vi "Match Block Upload Response.vi"(8 "error in":errorcluster, 10 "Frame Data":u8[](array[numeric]), 11 "Block Upload Initiate in":refnum<class "Block Upload Initiate Transfer.lvclass">) -> (0 "error out":errorcluster, 1 "SDO Result":T1={"Success"=FALSE, "SDO abort code"={"Null"=TRUE, "Value"=84082688}, "Data"={"Null"=TRUE, "Data"=[]}} {"SDO abort code"."Value" items=["Toggle bit not allowed"=84082688, "SDO protocol timed out"=84148224, "Client/server command specifier not valid or unknown"=84148225, "Invalid block size (block mode only)"=84148226, "Invalid sequence number (block mode only)"=84148227, "CRC error (block mode only)"=84148228, "Out of memory"=84148229, "Attempt to read a write only object"=100728833, "Attempt to write a read only object"=100728834, "Object does not exist in the object dictionary"=100794368, "Object cannot be mapped to the PDO"=100925505, "The number and length of the objects to be mapped would exceed PDO length"=100925506, "General parameter incompatibility reason"=100925507, "General internal incompatibility in the device"=100925511, "Access failed due to an hardware error"=101056512, "Data type does not match, length of service parameter does not match"=101122064, "Data type does not match, length of service parameter too high"=101122066, "Data type does not match, length of service parameter too low"=101122067, "Sub-index does not exist"=101253137, "Invalid value for parameter (download only)"=101253168, "Value of parameter written too high (download only)"=101253169, "Value of parameter written too low (download only)"=101253170, "Maximum value is less than minimum value"=101253174, "Resource not available: SDO connection"=101318691, "General error"=134217728, "Data cannot be transferred or stored to the application"=134217760, "Data cannot be transferred or stored to the application because of local control"=134217761, "Data cannot be transferred or stored to the application because of the present device stable"=134217762, "Object dictionary dynamic generation fails or no object dictionary is present (e.g. object dictionary is generated from file and generation fails because of an file error)"=134217763, "No data available"=134217764]; "Data"."Data" format="%02x"}, 2 "Match":bool, 3 "SDO Transfer out":refnum<class "SDO Transfer.lvclass">)   [LabVIEW 2020, in "CANopen.lvlib" / "SDO Manager.lvlib" / "Block Upload Initiate Transfer.lvclass"]
uses:
  Block Upload Initiate Transfer.lvclass
  Block Upload Initiate Transfer.lvclass/Block Upload Initiate Transfer.ctl
  D:/git/CANopen-LabVIEW/source/SDO Manager/SDO Manager/SDO Transfer/SDO Transfer.lvclass
  D:/git/CANopen-LabVIEW/source/Response Matcher/IResponse/IMatch Response.lvclass
  D:/git/CANopen-LabVIEW/source/SDO Manager/SDO Manager/Block Upload Initiate Transfer/Block Upload Initiate Transfer.lvclass
  Block Upload Sub-Block Transfer/Block Upload Sub-Block Transfer.lvclass
  D:/git/CANopen-LabVIEW/source/SDO Manager/SDO Manager/Block Upload Sub-Block Transfer/Block Upload Sub-Block Transfer.lvclass
  SDO Transfer/SDO Transfer.lvclass
  SDO Transfer/SDO abort code.ctl
  Typedefs/SDO Result.ctl
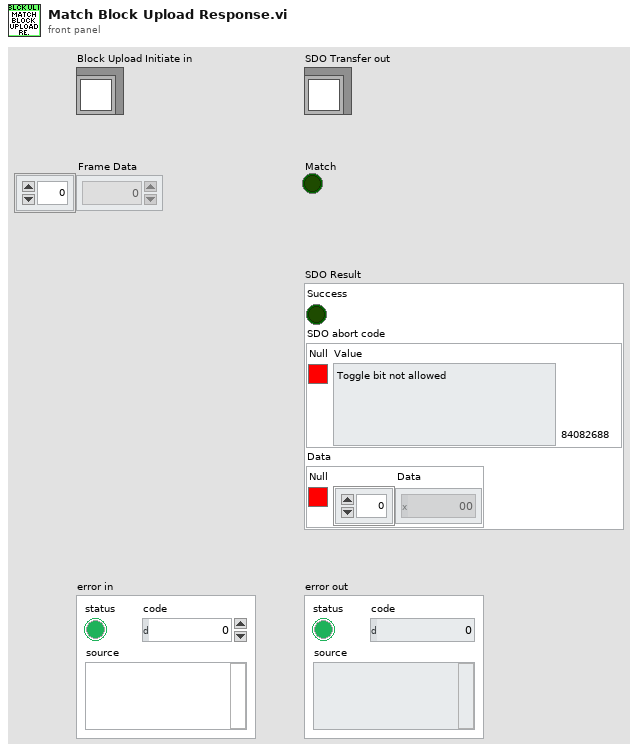
[diagram p1: front panel]
types:
  T1 = typedef "CANopen.lvlib/SDO Manager.lvlib/SDO Transfer.lvclass/SDO Result.ctl" = cluster{"Success":bool, "SDO abort code":cluster{"Null":bool, "Value":T2}, "Data":cluster{"Null":bool, "Data":u8[]}}
  T2 = typedef "CANopen.lvlib/SDO Manager.lvlib/SDO Transfer.lvclass/SDO abort code.ctl" = u32
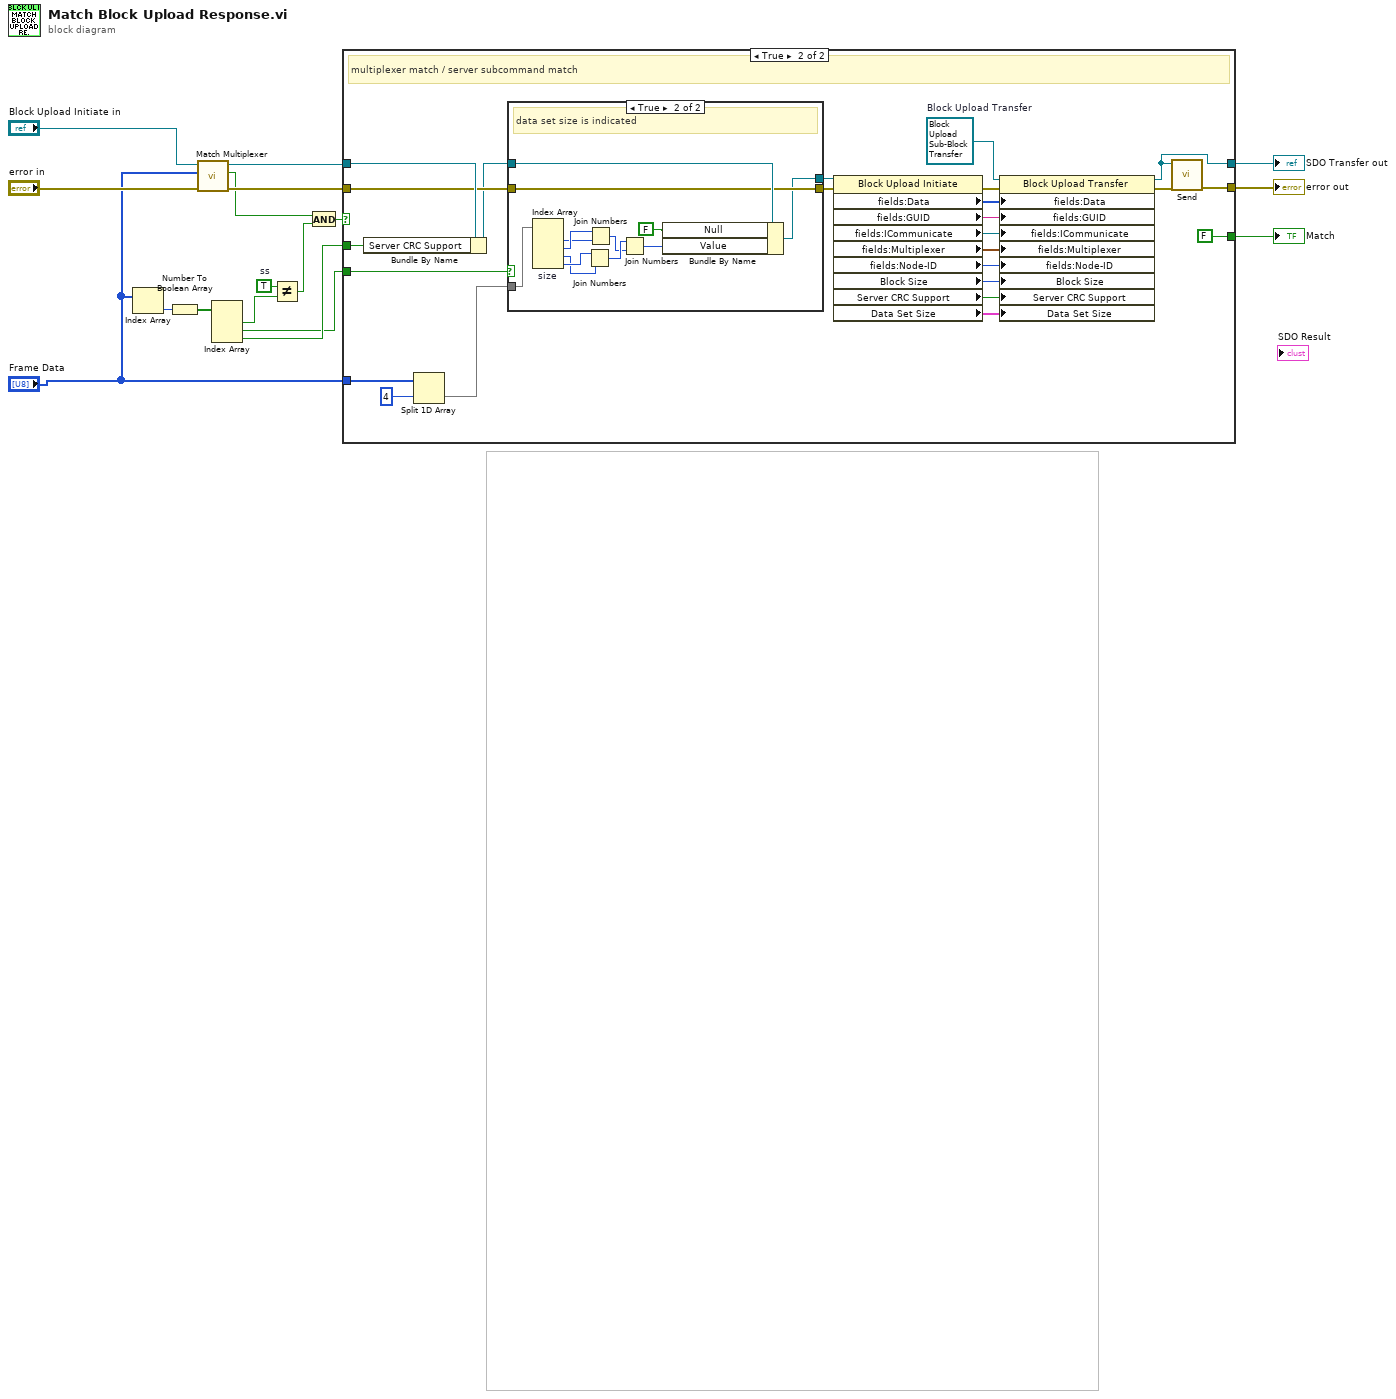
[diagram p0: block diagram]
diagram:
  w14 = TRUE  # ss
  n1 = Index Array(array="Frame Data") -> (element=w2:u8)  [unwired: 1 in]
  n2 = Number To Boolean Array(number=w2) -> (Boolean array=w12:bool[])
  n3 = call "Match Multiplexer.vi"("error in"="error in", "Frame Data"="Frame Data", "SDO Transfer in"="Block Upload Initiate in") -> ("error out"=w6:errorcluster, "Match"=w3:bool, "SDO Transfer out"=w4:refnum<class "Block Upload Initiate Transfer.lvclass">)  [unwired: 6 in]
  n4 = Index Array(array=w12) -> (element #1=w17:bool, element #2=w15:bool, element #3=w16:bool)  [unwired: 3 in]
  n5 = Not Equal?(x=w14, y=w17) -> (x != y?=w13:bool)
  n6 = And(x=w3, y=w13) -> (x .and. y?=w11:bool)
  n7 = case shown="True" w11 {
    tunnel: w6 -> [w19 w42]
    tunnel: w4 -> [w18 w43]
    tunnel: [w18 w20] -> w8
    tunnel: [w19 w28] -> w9
    tunnel: [_ FALSE] -> w10
    tunnel: w15 -> [_ w40]
    tunnel: w16 -> [_ w39]
    tunnel: "Frame Data" -> [_ w25]
    frame False {
      # "no match"
    }
    frame True {
      w37 = refnum<class "Block Upload Sub-Block Transfer.lvclass"> refnum  # Block Upload Transfer
      # "multiplexer match / server subcommand match"
      n8 = Bundle By Name(cluster=w43, "Server CRC Support"=w39) -> (w41:refnum<class "Block Upload Initiate Transfer.lvclass">)
      n9 = Split 1D Array(array=w25, index=4) -> (second subarray=w24:u8[])  [unwired: 1 out]
      n10 = case shown="True" w40 {
        tunnel: w24 -> [_ w55]
        tunnel: w41 -> [w44 w50]
        tunnel: w42 -> [w45 w48]
        tunnel: [w44 w47] -> w35
        tunnel: [w45 w48] -> w36
        frame False {
          # "data set size is not indicated"
        }
        frame True {
          # "data set size is indicated"
          n11 = Index Array "size"(array=w55) -> (element #1=w51:u8, element #2=w52:u8, element #3=w53:u8, element #4=w54:u8)  [unwired: 4 in]
          n12 = Join Numbers(hi=w54, lo=w53) -> ((hi.lo)=w57:u16)
          n13 = Join Numbers(hi=w52, lo=w51) -> ((hi.lo)=w56:u16)
          n14 = Join Numbers(hi=w57, lo=w56) -> ((hi.lo)=w46:u32)
          n15 = Bundle By Name(cluster=w50, "Null"=FALSE ("Data Set Size.Null"), "Value"=w46) -> (w47:refnum<class "Block Upload Initiate Transfer.lvclass">)
        }
      }
      n16 = property class="Block Upload Initiate"(reference=w35, error in=w36) -> (error out=w34:errorcluster, "fields:Data"=w22:u8[], "fields:GUID"=w30:string, "fields:ICommunicate"=w31:refnum<class "ICommunicate.lvclass">, "fields:Multiplexer"=w32:cluster{"Index":u16, "Sub-Index":u8}, "fields:Node-ID"=w33:u8, "Block Size"=w27:u8, "Server CRC Support"=w23:bool, "Data Set Size"=w21:cluster{"Null":bool, "Value":u32})  [unwired: 1 out]
      n17 = property class="Block Upload Transfer"(reference=w37, error in=w34, "fields:Data"=w22, "fields:GUID"=w30, "fields:ICommunicate"=w31, "fields:Multiplexer"=w32, "fields:Node-ID"=w33, "Block Size"=w27, "Server CRC Support"=w23, "Data Set Size"=w21) -> (reference out=w20:refnum<class "Block Upload Sub-Block Transfer.lvclass">, error out=w29:errorcluster)
      n18 = call-dynamic "Send.vi"("error in"=w29, "Block Upload Transfer in"=w20) -> ("error out"=w28:errorcluster)  [unwired: 9 in]
    }
  }
  "Match" <- w10
  "error out" <- w9
  "SDO Transfer out" <- w8
